vi "digital-on-off-delay-one-shot-test.vi"() -> ()   [LabVIEW 2019]
uses:
  <vilib>/Rock Robotics/WPI/ThirdParty/JAS_Junk/TrajLib/Trajectory_Library.lvlib
panel:
  in  "Tab Control":enum32{"Control Panel", "Logic"}(tab)
  in  "Input":bool
  out "On Delay\nOutput":bool
  in  "On Delay\nTime":dbl=10.0
  out "On Delay\nRemaining":dbl
  in  "Off Delay\nTime":dbl=3.0
  out "Off Delay\nOutput":bool
  out "Off Delay\nRemaining":dbl
  out "One Shot\nOutput":bool
  out "One Shot\nRemaining":dbl
  in  "One Shot\nTime":dbl=5.0
  out "Digital State Chart":cluster{dbl, dbl, dbl, dbl, dbl, dbl}(graph)
  # "ON DELAY, OFF DELAY,\nONE SHOT  TEST"
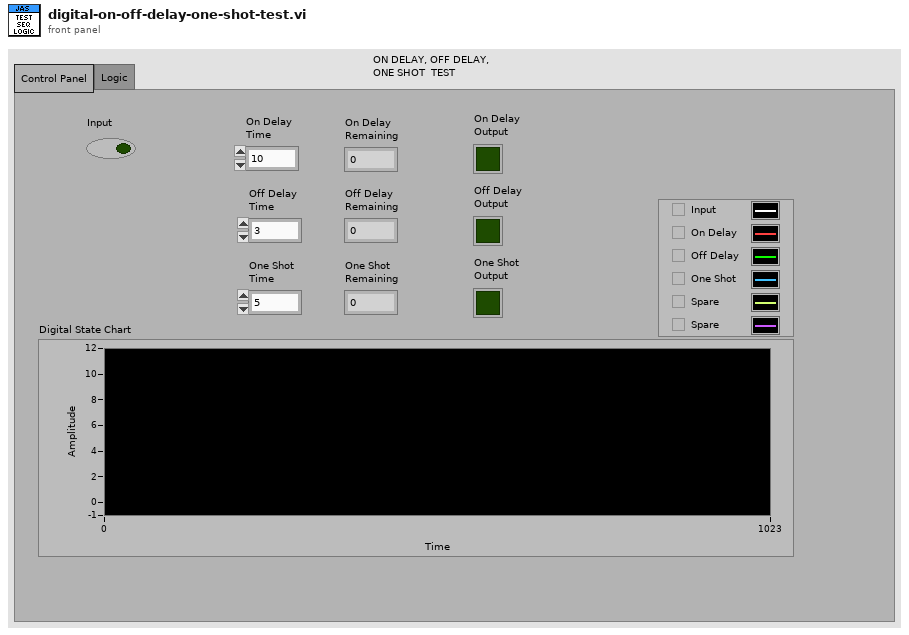
[diagram p1: front panel]
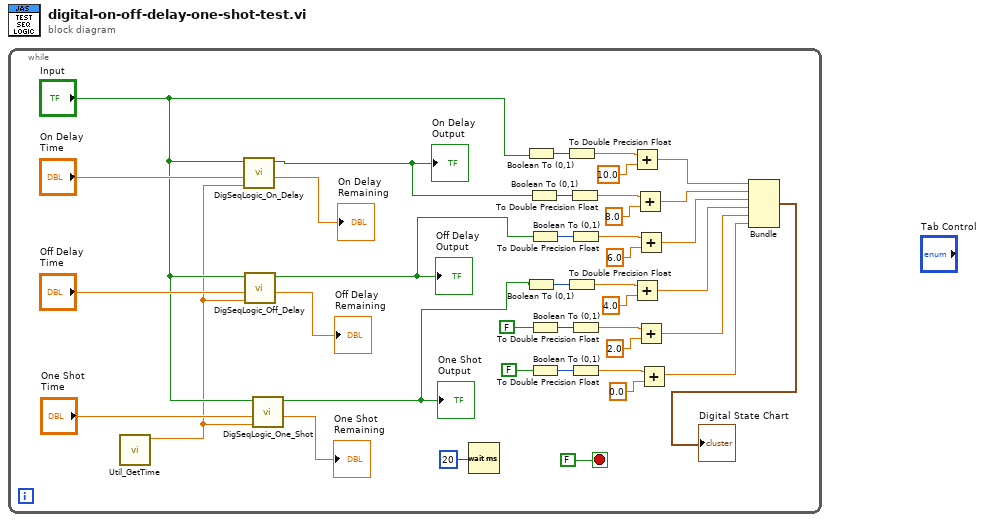
[diagram p0: block diagram]
diagram:
  n1 = while {
    stop <- FALSE stop-if-true
    n2 = call <vilib>:"Util_GetTime.vi"() -> ("FPGA_Time_Seconds"=w1:dbl)  [unwired: 10 in, 1 out]
    n3 = call <vilib>:"DigSeqLogic_On_Delay.vi"("Time"=w1, "Delay"="On Delay\nTime", "Input"="Input") -> ("Remain"=→"On Delay\nRemaining":dbl, "Output"=w5:bool)  [unwired: 7 in]
    "On Delay\nOutput" <- w5
    n4 = call <vilib>:"DigSeqLogic_Off_Delay.vi"("Time"=w1, "Delay"="Off Delay\nTime", "Input"="Input") -> ("Remain"=→"Off Delay\nRemaining":dbl, "Output"=w4:bool)  [unwired: 7 in]
    "Off Delay\nOutput" <- w4
    n5 = call <vilib>:"DigSeqLogic_One_Shot.vi"("Time"=w1, "OneShot"="One Shot\nTime", "Input"="Input") -> ("Remain"=→"One Shot\nRemaining":dbl, "Output"=w3:bool)  [unwired: 7 in]
    "One Shot\nOutput" <- w3
    n6 = Wait (ms)(milliseconds to wait=u32 20) -> ()  [unwired: 1 out]
    n7 = Boolean To (0,1)(Boolean="Input") -> (0, 1=w15:i16)
    n8 = Boolean To (0,1)(Boolean=w3) -> (0, 1=w16:i16)
    n9 = Boolean To (0,1)(Boolean=w5) -> (0, 1=w18:i16)
    n10 = Boolean To (0,1)(Boolean=w4) -> (0, 1=w20:i16)
    n11 = Boolean To (0,1)(Boolean=FALSE) -> (0, 1=w22:i16)
    n12 = Boolean To (0,1)(Boolean=FALSE) -> (0, 1=w24:i16)
    n13 = To Double Precision Float(number=w15) -> (double precision float=w31:dbl)
    n14 = To Double Precision Float(number=w16) -> (double precision float=w17:dbl)
    n15 = To Double Precision Float(number=w18) -> (double precision float=w19:dbl)
    n16 = To Double Precision Float(number=w20) -> (double precision float=w21:dbl)
    n17 = To Double Precision Float(number=w22) -> (double precision float=w23:dbl)
    n18 = To Double Precision Float(number=w24) -> (double precision float=w25:dbl)
    n19 = Add(x=w31, y=10.0) -> (x+y=w32:dbl)
    n20 = Add(x=w17, y=4.0) -> (x+y=w30:dbl)
    n21 = Add(x=w19, y=8.0) -> (x+y=w28:dbl)
    n22 = Add(x=w21, y=6.0) -> (x+y=w29:dbl)
    n23 = Add(x=w23, y=2.0) -> (x+y=w26:dbl)
    n24 = Add(x=w25, y=0.0) -> (x+y=w27:dbl)
    n25 = Bundle(w32, w28, w29, w30, w26, w27) -> (→"Digital State Chart":cluster{dbl, dbl, dbl, dbl, dbl, dbl})  [unwired: 1 in]
  }
